vi "forceBendtozero2.vi"(1 "data":dbl[](array[numeric])) -> (0 "forced data":dbl[](array[numeric]))   [LabVIEW 2015]
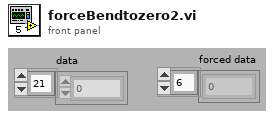
[diagram p1: front panel]
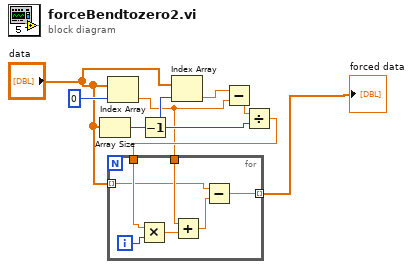
[diagram p0: block diagram]
diagram:
  n1 = Array Size(array="data") -> (size(s)=w8:i32)
  n2 = Index Array(array="data", index=0) -> (element=w3:dbl)
  n3 = Decrement(x=w8) -> (x-1=w5:i32)
  n4 = Index Array(array="data", index=w5) -> (element=w7:dbl)
  n5 = Subtract(x=w7, y=w3) -> (x-y=w6:dbl)
  n6 = Divide(x=w6, y=w5) -> (x/y=w4:dbl)
  n7 = for {
    tunnel: "data" -> [w11] mode=indexing
    tunnel: w4 -> [w15]
    tunnel: w3 -> [w13]
    tunnel: [w10] -> w1 mode=indexing
    i -> [w16]
    n8 = Multiply(x=w15, y=w16) -> (x*y=w14:dbl)
    n9 = Add(x=w13, y=w14) -> (x+y=w12:dbl)
    n10 = Subtract(x=w11, y=w12) -> (x-y=w10:dbl)
  }
  "forced data" <- w1
